vi "IBM4_Close.vi"(8 "error in":errorcluster, 11 "COM resource in":refnum<visa-resource-name>="COM3") -> (0 "error out":errorcluster)   [LabVIEW 2021, in "IBM4.lvlib"]
doc: "Close the IBM4"
uses:
  <instrlib>/IBM4/IBM4.lvlib
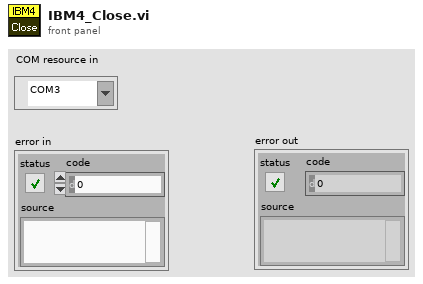
[diagram p1: front panel]
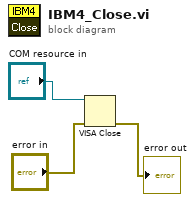
[diagram p0: block diagram]
diagram:
  n1 = VISA Close(VISA resource name="COM resource in", error in (no error)="error in") -> (error out=→"error out":errorcluster)
